vi "PCO_SetTriggerMode.vi"(8 "error in (no error)":errorcluster {"code" format="%x"}, 10 "wTriggerMode":u16(ring) items=["auto sequence"=0, "software trigger"=1, "external exposure start & software trigger"=2, "external exposure control"=3, "external synchronized"=4, "fast external exposure control"=5, "external CDS control"=6, "slow external exposure control"=7, "external synchronized HDSDI"=258], 11 "ph":u64) -> (0 "error out":errorcluster {"code" format="%x"}, 2 "ErrorMessage":i32 format="%x", 3 "ph out":u64)   [LabVIEW 2019, in "SDK.lvlib" / "TimingControl.lvlib"]
doc: "<b>Description:</b>\nThis function does set the trigger mode of the camera. For a short description of the available trigger modes, see table Explanation of available trigger modes.\nDetailed description of trigger and acquire modes can be found in the respective camera manual.\nIn all trigger modes effective image exposure depends also on the acquire mode settings and acquire signal input.\nThe command will be rejected, if Recording State is [run], see PCO_GetRecordingState.\n\n<b>Supported camera type:</b>\nAll cameras\n\n<b>Descriptor dependency:</b>\nNone"
uses:
  TimingControl.lvlib
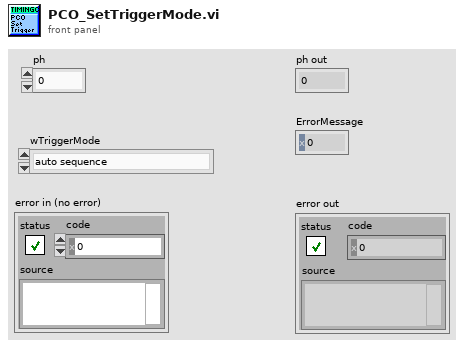
[diagram p1: front panel]
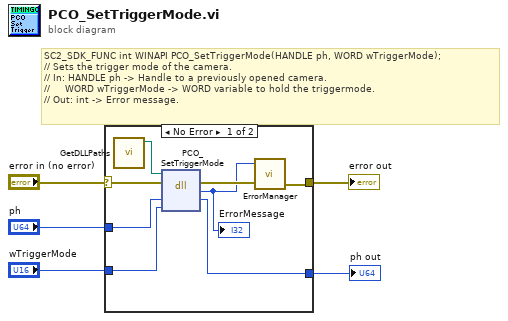
[diagram p0: block diagram]
diagram:
  # "SC2_SDK_FUNC int WINAPI PCO_SetTriggerMode(HANDLE ph, WORD wTriggerMode);\n// Sets the trigger mode of the camera.\n// In: HANDLE ph -> Handle to a previously opened camera.\n//     WORD wTriggerMode -> WORD variable to hold the triggermode.\n// Out: int -> Error message."
  n1 = case shown="No Error" "error in (no error)" {
    selector: "error in (no error)" -> [w10 w15]
    tunnel: "ph" -> [w13 w14]
    tunnel: [w12 w14] -> w4
    tunnel: "wTriggerMode" -> [w11 _]
    tunnel: [w8 w15] -> w3
    frame No Error {
      n2 = call "GetDLLPaths.vi"() -> ("SC2_Cam_Path"=w6:path)  [unwired: 9 in, 2 out]
      n3 = dll-call lib="?" fn="PCO_SetTriggerMode"(path in=w6, error in=w10, "ph"=w13, "wTriggerMode"=w11) -> (error out=w9:errorcluster, "return type"=w7:i32, "ph"=w12:u64)  [unwired: 2 in, 1 out]
      "ErrorMessage" <- w7
      n4 = call "ErrorManager.vi"("error in (no error)"=w9, "error code"=w7) -> ("error out"=w8:errorcluster)  [unwired: 3 in]
    }
    frame Error {
    }
  }
  "ph out" <- w4
  "error out" <- w3
